vi "Read Measurement.vi"(8 "error in":errorcluster, 10 "call id":T1, 11 "gRPCid in":T1) -> (0 "error out":errorcluster, 1 "measure success?":bool, 2 "measurement results":T2, 3 "gRPCid out":T1)   [LabVIEW 2025, in "Automotive-Ethernet_LabVIEW.lvlib"]
doc: "Read and unpack the measurement results, until the measurement fails."
uses:
  Automotive-Ethernet_LabVIEW.lvlib
  <vilib>/gRPC/LabVIEW gRPC Library/Shared/grpcId.ctl
  controls/Measurement Results.ctl
  34829905-00c5-4e32-9a4f-e87a22ec28de.vi
  <vilib>/gRPC/LabVIEW gRPC Library/Server API/Translate Protobuf Error.vi
  <vilib>/AdvancedString/1D String Array to Delimited String.vi
  <vilib>/gRPC/LabVIEW gRPC Library/Server API/Server/Get Server DLL Path.vi
  <vilib>/gRPC/Generated APIs/ni/measurementlink/measurement/v2/Measurement Service Client V2/Measurement Service Client V2.lvlib
  <vilib>/gRPC/LabVIEW gRPC Library/grpc-lvsupport-release.lvlib
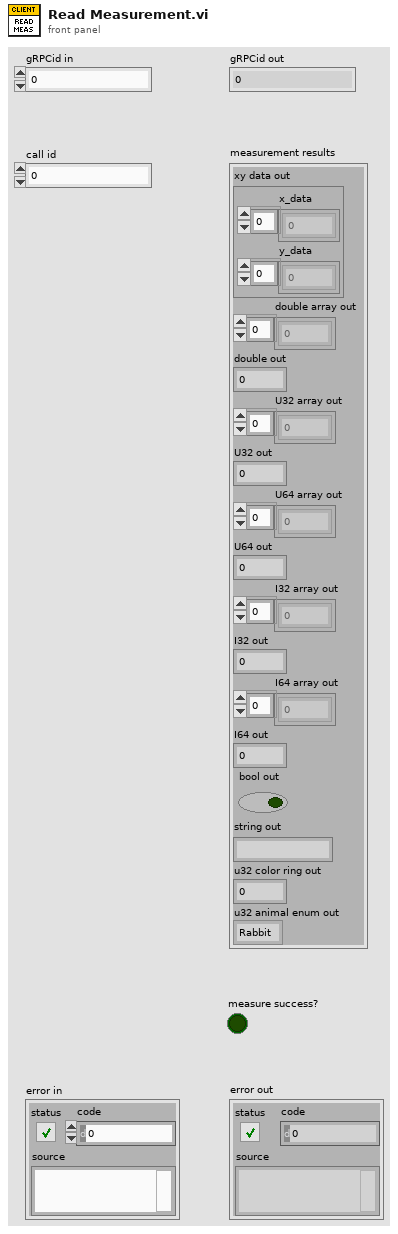
[diagram p1: front panel]
types:
  T1 = typedef "grpc-lvsupport-release.lvlib/grpcId.ctl" = u64
  T2 = typedef "Automotive-Ethernet_LabVIEW.lvlib/Measurement Results.ctl" = cluster{"xy data out":cluster{"x_data":dbl[], "y_data":dbl[]}, "double array out":dbl[], "double out":dbl, "U32 array out":u32[], "U32 out":u32, "U64 array out":u64[], "U64 out":u64, "I32 array out":i32[], "I32 out":i32, "I64 array out":i64[], "I64 out":i64, "bool out":bool, "string out":string, "u32 color ring out":u32, "u32 animal enum out":enum32{"Rabbit", "Gopher", "Badger"}}
  T3 = typedef "Measurement Service Client V2.lvlib/ni_measurementlink_measurement_v2_MeasureResponse.ctl" = cluster{"outputs":T4}
  T4 = typedef "Measurement Service Client V2.lvlib/google_protobuf_Any.ctl" = cluster{"type_url":string, "value":u8[]}
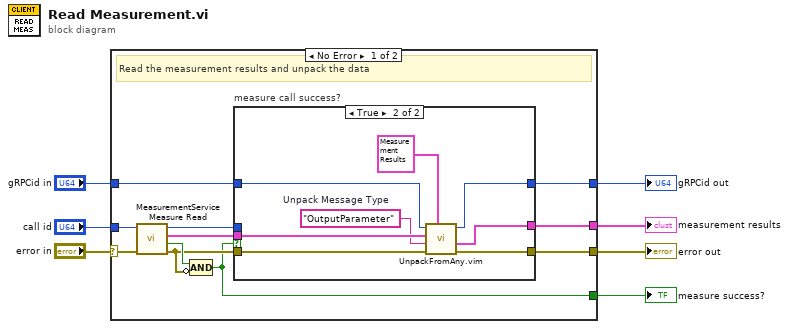
[diagram p0: block diagram]
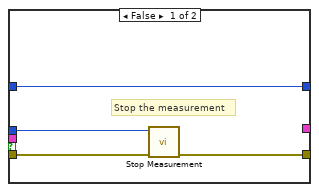
[diagram p2: hidden frame]
diagram:
  n1 = case shown="No Error" "error in" {
    selector: "error in" -> [w15 w31]
    tunnel: "gRPCid in" -> [w17 w32]
    tunnel: "call id" -> [w16 _]
    tunnel: [w14 _] -> w4
    tunnel: [w13 w32] -> w3
    tunnel: [w11 w31] -> w2
    tunnel: [w8 _] -> w1
    frame No Error {
      # "Read the measurement results and unpack the data"
      n2 = call <vilib>:"MeasurementService Measure Read.vi"("error in"=w15, "Call ID in"=w16) -> ("error out"=w9:errorcluster, "Success"=w10:bool, "Response Data"=w12:T3, "Call ID"=w18:T1)  [unwired: 6 in]
      n3 = Compound Arithmetic op=AND(w10, invert w9) -> (w8:bool)
      n4 = case "measure call success?" shown="True" w8 {
        tunnel: w12 -> [_ w30]
        tunnel: [w20 w29] -> w11
        tunnel: w9 -> [w21 w28]
        tunnel: [w22 w26] -> w13
        tunnel: [_ w24] -> w14
        tunnel: w17 -> [w22 w23]
        tunnel: w18 -> [w19 _]
        frame False {
          # "Stop the measurement"
          n5 = call "Stop Measurement.vi"("error in"=w21, "call id"=w19) -> ("error out"=w20:errorcluster)  [unwired: 9 in]
        }
        frame True {
          w25 = "OutputParameter"  # Unpack Message Type
          n6 = call "UnpackFromAny.vim"("Data Type"=T2 {"xy data out"={"x_data"=[], "y_data"=[]}, "double array out"=[], "double out"=0.0, "U32 array out"=[], "U32 out"=0, "U64 array out"=[], "U64 out"=0, "I32 array out"=[], "I32 out"=0, "I64 array out"=[], "I64 out"=0, "bool out"=FALSE, "string out"="", "u32 color ring out"=0, "u32 animal enum out"=enum."Rabbit"} ("measurement results"), "error in"=w28, "Message Type"=w25, "Any"=w30, "gRPCid in"=w23) -> ("error out"=w29:errorcluster, "Unpacked Value"=w24:T2, "gRPCid out"=w26:u64)  [unwired: 4 in]
        }
      }
    }
    frame Error {
      # "Pass"
    }
  }
  "measurement results" <- w4
  "gRPCid out" <- w3
  "error out" <- w2
  "measure success?" <- w1
